vi "barcode trail.vi"() -> ()   [LabVIEW 2015]
panel:
  out "error out":errorcluster
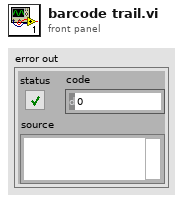
[diagram p1: front panel]
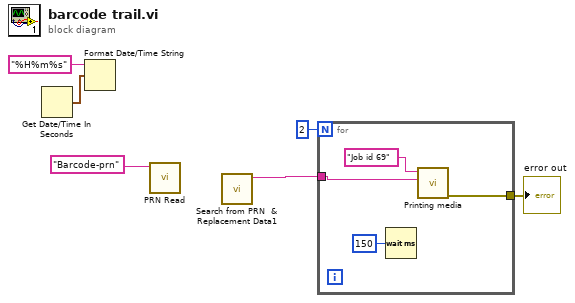
[diagram p0: block diagram]
diagram:
  n1 = Get Date/Time In Seconds() -> (seconds since 1Jan1904=w3:timestamp)
  n2 = Format Date/Time String(time format string (%c)="%H%m%s", seconds (now)=w3) -> ()  [unwired: 1 in, 1 out]
  n3 = call "PRN Read.vi"("prn"="Barcode-prn") -> ()  [unwired: 9 in, 2 out]
  n4 = call "Search from PRN  & Replacement Data1.vi"() -> ("send on  barcode printer"=w5:string)  [unwired: 9 in, 1 out]
  n5 = for {
    N: 2 -> [_]
    tunnel: w5 -> [w10]
    tunnel: [w7] -> w1
    n6 = Wait (ms)(milliseconds to wait=u32 150) -> ()  [unwired: 1 out]
    n7 = call "Printing media.vi"("send on  barcode printer"=w10, "printer name"="Job id 69") -> ("error out"=w7:errorcluster)  [unwired: 9 in]
  }
  "error out" <- w1
